vi "init.vi"(8 "error in":errorcluster, 10 "TBM module configuration in":refnum<class "TBM module configuration.lvclass">, 11 "tag bus configurable plugin module in":refnum<class "TEST RUNTIME.lvclass">) -> (0 "error out":errorcluster, 1 "data allocations":T1, 2 "execution settings":T4, 3 "tag bus configurable plugin module out":refnum<class "TEST RUNTIME.lvclass">)   [LabVIEW 2013, in "configuration tests.lvlib" / "TEST RUNTIME.lvclass"]
doc: "Provides an interface for initializing a module at runtime. While this interface performs no operations, a child should provide an override which may open any necessary references or sessions, allocate necessary memory, and perform any final configuration validataion before providing the full configuration <b>execution data</b> to the calling process."
uses:
  TEST RUNTIME.lvclass
  <vilib>/NI/Tag Bus Module Framework/module configuration/TBM module configuration.lvclass
  <vilib>/NI/Tag Bus Module Framework/runtime/execution settings.ctl
  <vilib>/NI/Tag Bus Module Framework/channel/data tables.ctl
  <vilib>/NI/Tag Bus/dictionary/data dictionary.lvclass
  <vilib>/NI/Tag Bus/dictionary table pair.ctl
  <vilib>/NI/Tag Bus/table/data table.ctl
  configuration/TEST CONFIGURATION.lvclass
  state control.ctl
  configuration/TEST CONFIGURATION.lvclass/TEST CONFIGURATION.ctl
  <vilib>/NI/Tag Bus/tag/tag descriptor.lvclass/tag descriptor.ctl
  <vilib>/NI/Tag Bus/dictionary/data dictionary.lvclass/data dictionary.ctl
  control module.ctl
  TEST RUNTIME.lvclass/TEST RUNTIME.ctl
  <vilib>/NI/Tag Bus/dictionary/lookup polymorphs/locate double.vi
  <vilib>/NI/Tag Bus/tag/read tag name.vi
  configuration/Read state module configuration.vi
  configuration/Read control functions.vi
  <vilib>/NI/Tag Bus/dictionary/search/find data index.vi
  <vilib>/NI/Tag Bus/dictionary/search/search string list.vi
  <vilib>/NI/Tag Bus/dictionary/tag not found.vi
  <vilib>/NI/Tag Bus Module Framework/channel/TBM channel.lvclass
  <vilib>/NI/Tag Bus Module Framework/runtime/TBM module execution interface.lvclass
  <vilib>/NI/Tag Bus/tag bus.lvlib
  <vilib>/NI/Tag Bus/table/data table.lvlib
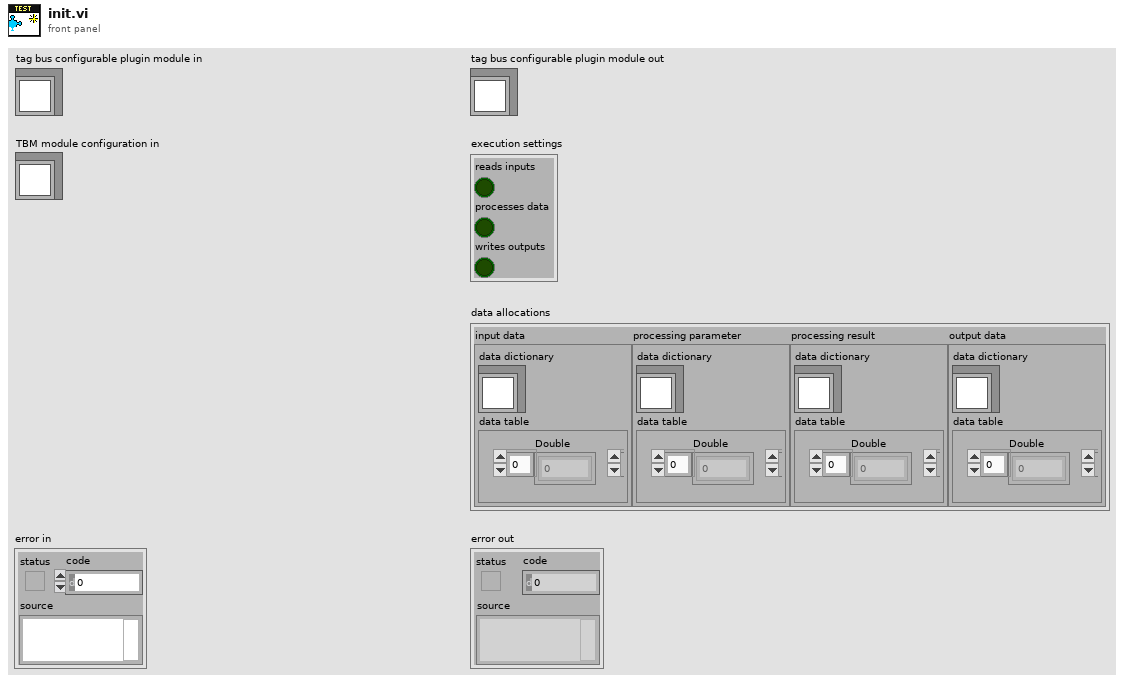
[diagram p1: front panel]
types:
  T1 = typedef "TBM channel.lvclass/data tables.ctl" = cluster{"input data":T2, "processing parameter":T2, "processing result":T2, "output data":T2}
  T2 = typedef "tag bus.lvlib/dictionary table pair.ctl" = cluster{"data dictionary":refnum<class "data dictionary.lvclass">, "data table":T3}
  T3 = typedef "tag bus.lvlib/data table.lvlib/data table.ctl" = cluster{"Double":dbl[], "Single":sgl[], "I64":i64[], "I32":i32[], "I16":i16[], "I8":i8[], "U64":u64[], "U32":u32[], "U16":u16[], "U8":u8[], "Boolean":bool[], "String":string[], "Array of Double":cluster{"DBL Array":dbl[]}[], "Array of Single":cluster{"SGL Array":sgl[]}[], "Array of I64":cluster{"I64 Array":i64[]}[], "Array of I32":cluster{"I32 Array":i32[]}[], "Array of I16":cluster{"I16 Array":i16[]}[], "Array of I8":cluster{"I8 Array":i8[]}[], "Array of U64":cluster{"U64 Array":u64[]}[], "Array of U32":cluster{"U32 Array":u32[]}[], "Array of U16":cluster{"U16 Array":u16[]}[], "Array of U8":cluster{"U8 Array":u8[]}[], "Array of Boolean":cluster{"Boolean Array":bool[]}[], "Array of String":cluster{"String Array":string[]}[]}
  T4 = typedef "TBM module execution interface.lvclass/execution settings.ctl" = cluster{"reads inputs":bool, "processes data":bool, "writes outputs":bool}
  T5 = typedef "configuration tests.lvlib/TEST RUNTIME.lvclass/state control.ctl" = cluster{"state":u8, "control index (dbl)":i32, "output index (dbl)":i32}
  T6 = typedef "configuration tests.lvlib/TEST RUNTIME.lvclass/control module.ctl" = cluster{"setpoint index (dbl)":i32, "proc var index (dbl)":i32, "output index (dbl)":i32, "output range":cluster{"output high":dbl, "output low":dbl}, "Kp":dbl, "Ki":dbl, "Kd":dbl, "error int":dbl, "last error":dbl}
  T7 = typedef "user tag bus module configuration.lvclass/state module configuration.ctl" = cluster{"fixed input":refnum<class "TBM channel.lvclass">, "fixed output":refnum<class "TBM channel.lvclass">, "initial state":u8}
  T8 = typedef "user tag bus module configuration.lvclass/control module configuration.ctl" = cluster{"name":string, "setpoint":refnum<class "TBM channel.lvclass">, "process variable":refnum<class "TBM channel.lvclass">, "output":refnum<class "TBM channel.lvclass">, "gains":T9, "output range":cluster{"output high":dbl, "output low":dbl}}
  T9 = typedef "user tag bus module configuration.lvclass/gains.ctl" = cluster{"Kp":dbl, "Ki":dbl, "Kd":dbl}
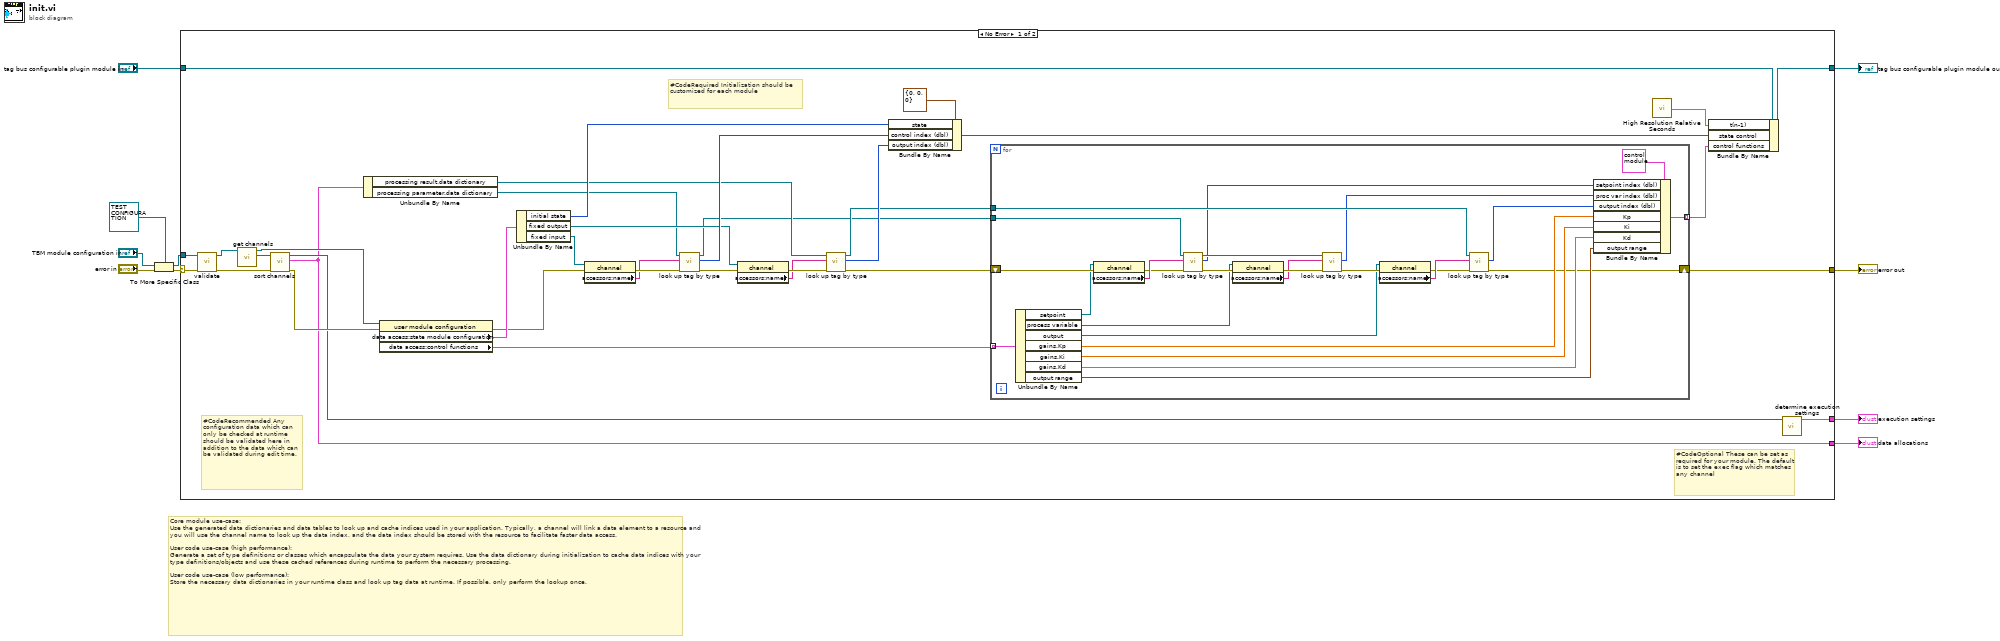
[diagram p0: block diagram]
diagram:
  # "Core module use-case:\nUse the generated data dictionaries and data tables to look up and cache indices used in your application. Typically, a channel will link a data element to a resource and you will use the channel name to look up the data index, and the data index should be stored with the resource to facilitate faster data access.\n\nUser code use-case (high performance):\nGenerate a set of type definitions or classes which encapsulate the data your system requires. Use the data dictionary during initialization to cache data indices with your type definitions/objects and use these cached references during runtime to perform the necessary processing.\n\nUser code use-case (low performance):\nStore the necessary data dictionaries in your runtime class and look up tag data at runtime. If possible, only perform the lookup once."
  n1 = To More Specific Class(target class=refnum<class "TEST CONFIGURATION.lvclass"> refnum ("Synchronous module configuration"), reference="TBM module configuration in", error in="error in") -> (specific class reference=w9:refnum<class "TEST CONFIGURATION.lvclass">, error out=w10:errorcluster)
  n2 = case shown="No Error" w10 {
    selector: w10 -> [w40 w72]
    tunnel: w9 -> [w39 _]
    tunnel: "tag bus configurable plugin module in" -> [w45 w73]
    tunnel: [w34 w73] -> w4
    tunnel: [w14 w72] -> w3
    tunnel: [w35 _] -> w1
    tunnel: [w43 _] -> w2
    frame No Error {
      # "#CodeRecommended Any configuration data which can only be checked at runtime should be validated here in addition to the data which can be validated during edit time."
      # "#CodeOptional These can be set as required for your module. The default is to set the exec flag which matches any channel"
      # "#CodeRequired Initialization should be customized for each module"
      n3 = call-dynamic "validate.vi"("error in"=w40, "tag bus configurable plugin module configuration in"=w39) -> ("error out"=w41:errorcluster, "tag bus configurable plugin module configuration out"=w38:refnum<class "TEST CONFIGURATION.lvclass">)  [unwired: 8 in]
      n4 = call-dynamic "get channels.vi"("user tag bus module configuration In"=w38) -> ("channels"=w37:refnum<class "TBM channel.lvclass">[], "user tag bus module configuration Out"=w36:refnum<class "TEST CONFIGURATION.lvclass">)  [unwired: 9 in]
      n5 = call <vilib>:"sort channels.vi"("error in"=w41, "channels in"=w37) -> ("error out"=w44:errorcluster, "data allocations"=w35:T1, "channels out"=w42:refnum<class "TBM channel.lvclass">[])  [unwired: 7 in]
      n6 = Unbundle By Name(w35) -> ("processing result.data dictionary"=w18:refnum<class "data dictionary.lvclass">, "processing parameter.data dictionary"=w19:refnum<class "data dictionary.lvclass">)
      n7 = property class="user module configuration"(reference=w36, error in=w44) -> (error out=w29:errorcluster, "data access:state module configuration"=w33:T7, "data access:control functions"=w17:T8[])  [unwired: 1 out]
      n8 = Unbundle By Name(w33) -> ("initial state"=w31:u8, "fixed output"=w23:refnum<class "TBM channel.lvclass">, "fixed input"=w21:refnum<class "TBM channel.lvclass">)
      n9 = property class="channel"(reference=w21, error in=w29) -> (error out=w24:errorcluster, "accessors:name"=w20:string)  [unwired: 1 out]
      n10 = call-poly <vilib>:"look up tag by type.vi"("error in"=w24, "name"=w20, "data dictionary in"=w19) -> ("error out"=w28:errorcluster, "index"=w26:i32, "data dictionary out"=w12:refnum<class "data dictionary.lvclass">)  [unwired: 6 in]
      n11 = property class="channel"(reference=w23, error in=w28) -> (error out=w25:errorcluster, "accessors:name"=w22:string)  [unwired: 1 out]
      n12 = call-poly <vilib>:"look up tag by type.vi"("error in"=w25, "name"=w22, "data dictionary in"=w18) -> ("error out"=w15:errorcluster, "index"=w27:i32, "data dictionary out"=w13:refnum<class "data dictionary.lvclass">)  [unwired: 6 in]
      n13 = Bundle By Name(cluster=T5 {"state"=0, "control index (dbl)"=0, "output index (dbl)"=0} ("state control"), "state"=w31, "control index (dbl)"=w26, "output index (dbl)"=w27) -> (w30:T5)
      n14 = for {
        tunnel: w17 -> [w69] mode=indexing
        tunnel: [w70] -> w16 mode=indexing
        shift-right: [w55] -> w14
        shift-left: w15 -> [w58]
        tunnel: w13 -> [w52]
        tunnel: w12 -> [w51]
        n15 = Unbundle By Name(w69) -> ("setpoint"=w46:refnum<class "TBM channel.lvclass">, "process variable"=w47:refnum<class "TBM channel.lvclass">, "output"=w54:refnum<class "TBM channel.lvclass">, "gains.Kp"=w65:dbl, "gains.Ki"=w66:dbl, "gains.Kd"=w67:dbl, "output range"=w68:cluster{"output high":dbl, "output low":dbl})
        n16 = property class="channel"(reference=w46, error in=w58) -> (error out=w63:errorcluster, "accessors:name"=w64:string)  [unwired: 1 out]
        n17 = call-poly <vilib>:"look up tag by type.vi"("error in"=w63, "name"=w64, "data dictionary in"=w51) -> ("error out"=w57:errorcluster, "index"=w48:i32, "data dictionary out"=w50:refnum<class "data dictionary.lvclass">)  [unwired: 6 in]
        n18 = property class="channel"(reference=w47, error in=w57) -> (error out=w62:errorcluster, "accessors:name"=w61:string)  [unwired: 1 out]
        n19 = call-poly <vilib>:"look up tag by type.vi"("error in"=w62, "name"=w61, "data dictionary in"=w50) -> ("error out"=w56:errorcluster, "index"=w49:i32)  [unwired: 6 in, 1 out]
        n20 = property class="channel"(reference=w54, error in=w56) -> (error out=w59:errorcluster, "accessors:name"=w60:string)  [unwired: 1 out]
        n21 = call-poly <vilib>:"look up tag by type.vi"("error in"=w59, "name"=w60, "data dictionary in"=w52) -> ("error out"=w55:errorcluster, "index"=w53:i32)  [unwired: 6 in, 1 out]
        n22 = Bundle By Name(cluster=T6 {"setpoint index (dbl)"=0, "proc var index (dbl)"=0, "output index (dbl)"=0, "output range"={"output high"=100.0, "output low"=-100.0}, "Kp"=0.0, "Ki"=0.0, "Kd"=0.0, "error int"=0.0, "last error"=0.0} ("sample control module"), "setpoint index (dbl)"=w48, "proc var index (dbl)"=w49, "output index (dbl)"=w53, "Kp"=w65, "Ki"=w66, "Kd"=w67, "output range"=w68) -> (w70:T6)
      }
      n23 = call <vilib>:"High Resolution Relative Seconds.vi"() -> ("relative seconds"=w11:dbl)
      n24 = Bundle By Name(cluster=w45, "t(n-1)"=w11, "state control"=w30, "control functions"=w16) -> (w34:refnum<class "TEST RUNTIME.lvclass">)
      n25 = call <vilib>:"determine execution settings.vi"("channels"=w42) -> ("execution settings"=w43:T4)  [unwired: 10 in]
    }
    frame Error {
    }
  }
  "error out" <- w3
  "tag bus configurable plugin module out" <- w4
  "execution settings" <- w2
  "data allocations" <- w1
